vi "3c. Main.vi"() -> ()   [LabVIEW 2013]
uses:
  src/LabVIEW/LQ Core/QSize.ctl
  src/LabVIEW/Qt Widgets/QBoxLayout/Direction.ctl
  src/LabVIEW/LQ Core/LQCoreEngine/_Polymorphic Instances/Connect_CallbackIn_DBL.vi
  src/LabVIEW/Qt Widgets/QWidget/resize.vi
  src/LabVIEW/Qt Widgets/QWidget/setVisible.vi
  src/LabVIEW/LQ Core/LQCoreEngine/LQCoreEngine.lvclass
  src/LabVIEW/Qt Widgets/QLCDNumber/QLCDNumber.lvclass
  src/LabVIEW/Qwt/QwtSlider/QwtSlider.lvclass
  src/LabVIEW/Qt Widgets/QWidget/QWidget.lvclass
  src/LabVIEW/Qt Widgets/QBoxLayout/QBoxLayout.lvclass
panel:
  in  "Stop Button":bool
  # "Prerequisite knowledge/experience\n- Example 2. Managing a Widget Layout\n- Connector pane patterns\n\n\nDescription\nSignals are similar to Events or Notifications. Signals are handled by slots.\n\nExamples 3a, 3b and 3c show different ways of doing the same thing:  They listen for the signal that\nis emitted when you drag the slider in 2. Managing a Widget Layout, and then they use that signal\nto update the LCD.\n\nThis example uses a callback VI to connect the slider to the LCD.\n\n\nShowcase\n- Event-driven programming for widgets"
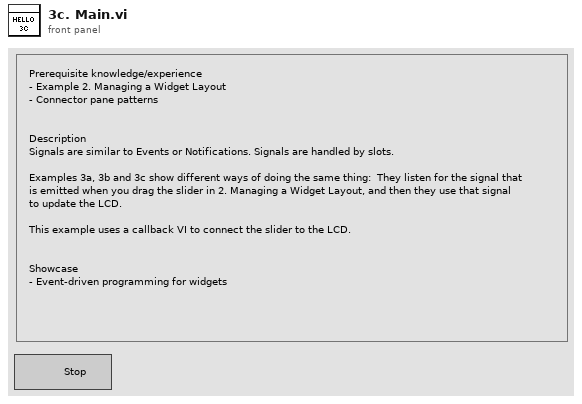
[diagram p1: front panel]
types:
  T1 = typedef "QBoxLayout.lvclass/Direction.ctl" = i32
  T2 = typedef "QSize.ctl" = cluster{"width":i32, "height":i32}
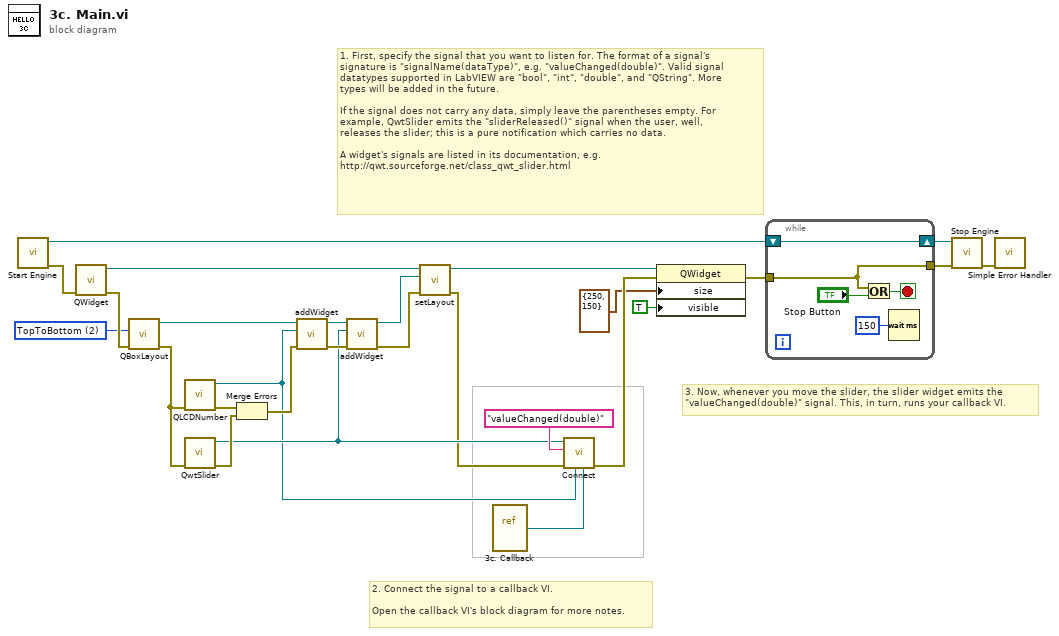
[diagram p0: block diagram]
diagram:
  w7 = T1 2 items=["LeftToRight", "RightToLeft", "TopToBottom", "BottomToTop"] ("direction")
  # "3. Now, whenever you move the slider, the slider widget emits the\n\"valueChanged(double)\" signal. This, in turn, runs your callback VI."
  # "1. First, specify the signal that you want to listen for. The format of a signal's\nsignature is \"signalName(dataType)\", e.g. \"valueChanged(double)\". Valid signal\ndatatypes supported in LabVIEW are \"bool\", \"int\", \"double\", and \"QString\". More\ntypes will be added in the future.\n\nIf the signal does not carry any data, simply leave the parentheses empty. For\nexample, QwtSlider emits the \"sliderReleased()\" signal when the user, well,\nreleases the slider; this is a pure notification which carries no data.\n\nA widget's signals are listed in its documentation, e.g.\nhttp://qwt.sourceforge.net/class_qwt_slider.html"
  # "2. Connect the signal to a callback VI.\n\nOpen the callback VI's block diagram for more notes."
  n1 = call "Start Engine.vi"() -> ("Error Out"=w21:errorcluster, "New Engine"=w5:refnum<class "LQCoreEngine.lvclass">)  [unwired: 10 in]
  n2 = call "QWidget.vi"("Error In"=w21) -> ("Error Out"=w20:errorcluster, "New QWidget"=w13:refnum<class "QWidget.lvclass">)  [unwired: 9 in]
  n3 = call "QBoxLayout.vi"("Error In"=w20, "direction"=w7) -> ("Error Out"=w19:errorcluster, "New QBoxLayout"=w18:refnum<class "QBoxLayout.lvclass">)  [unwired: 8 in]
  n4 = call "QLCDNumber.vi"("Error In"=w19) -> ("Error Out"=w16:errorcluster, "New QLCDNumber"=w6:refnum<class "QLCDNumber.lvclass">)  [unwired: 9 in]
  n5 = call "QwtSlider.vi"("Error In"=w19) -> ("Error Out"=w17:errorcluster, "New QwtSlider"=w10:refnum<class "QwtSlider.lvclass">)  [unwired: 9 in]
  n6 = Merge Errors(w16, w17) -> (w22:errorcluster)
  n7 = call "addWidget.vi"("Error In"=w22, "widget"=w6, "QBoxLayout In"=w18) -> ("Error Out"=w14:errorcluster, "QBoxLayout Out"=w15:refnum<class "QBoxLayout.lvclass">)  [unwired: 7 in]
  n8 = call "addWidget.vi"("Error In"=w14, "widget"=w10, "QBoxLayout In"=w15) -> ("Error Out"=w11:errorcluster, "QBoxLayout Out"=w12:refnum<class "QBoxLayout.lvclass">)  [unwired: 7 in]
  n9 = call "setLayout.vi"("Error In"=w11, "layout"=w12, "QWidget In"=w13) -> ("Error Out"=w8:errorcluster, "QWidget Out"=w9:refnum<class "QWidget.lvclass">)  [unwired: 7 in]
  n10 = vi-ref "3c. Callback.vi"() -> (w1:refnum<vi>)
  n11 = call-poly "Connect.vi"("Slot VI"=w1, "Receiver"=w6, "Error In"=w8, "Signal"="valueChanged(double)" ("Signal Signature"), "Sender In"=w10) -> ("Error Out"=w27:errorcluster)  [unwired: 5 in, 1 out]
  n12 = property class="QWidget"(reference=w9, error in=w27, "size"=T2 {"width"=250, "height"=150}, "visible"=TRUE) -> (error out=w4:errorcluster)  [unwired: 1 out]
  n13 = while {
    shift-right: [w32] -> w2
    shift-left: w5 -> [w32]
    tunnel: w4 -> [w29]
    tunnel: [w29] -> w3
    stop <- w30 stop-if-true
    n14 = Or(x=w29, y="Stop Button") -> (x .or. y?=w30:bool)
    n15 = Wait (ms)(milliseconds to wait=u32 150) -> ()  [unwired: 1 out]
  }
  n16 = call "Stop Engine.vi"("Error In"=w3, "LQCoreEngine"=w2) -> ("Error Out"=w25:errorcluster)  [unwired: 9 in]
  n17 = call <vilib>:"Simple Error Handler.vi"("error in (no error)"=w25) -> ()  [unwired: 4 in, 5 out]
